vi "CreateImages.vi"(8 "error in (no error)":errorcluster) -> (0 "error out":errorcluster, 3 "Images":T1)   [LabVIEW 2015]
uses:
  controls/Images.ctl
  <vilib>/vision/Image Controls.llb/IMAQ Image.ctl
  <vilib>/vision/NI_Vision_Development_Module.lvlib
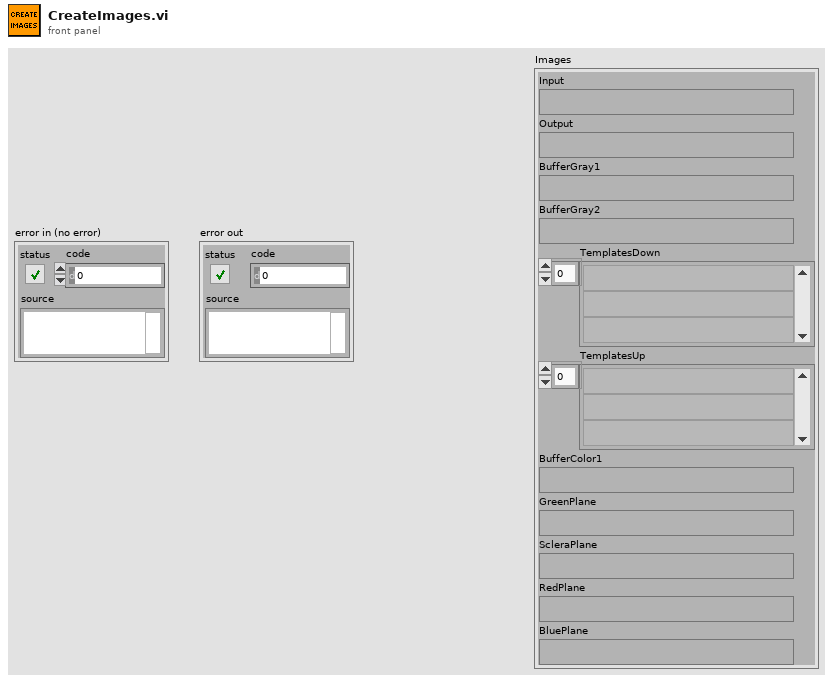
[diagram p1: front panel]
types:
  T1 = typedef "Images.ctl" = cluster{"Input":T2, "Output":T2, "BufferGray1":T2, "BufferGray2":T2, "TemplatesDown":T2[], "TemplatesUp":T2[], "BufferColor1":T2, "GreenPlane":T2, "ScleraPlane":T2, "RedPlane":T2, "BluePlane":T2}
  T2 = typedef "IMAQ Image.ctl" = refnum<image>
  T3 = typedef "Image Type" = u32
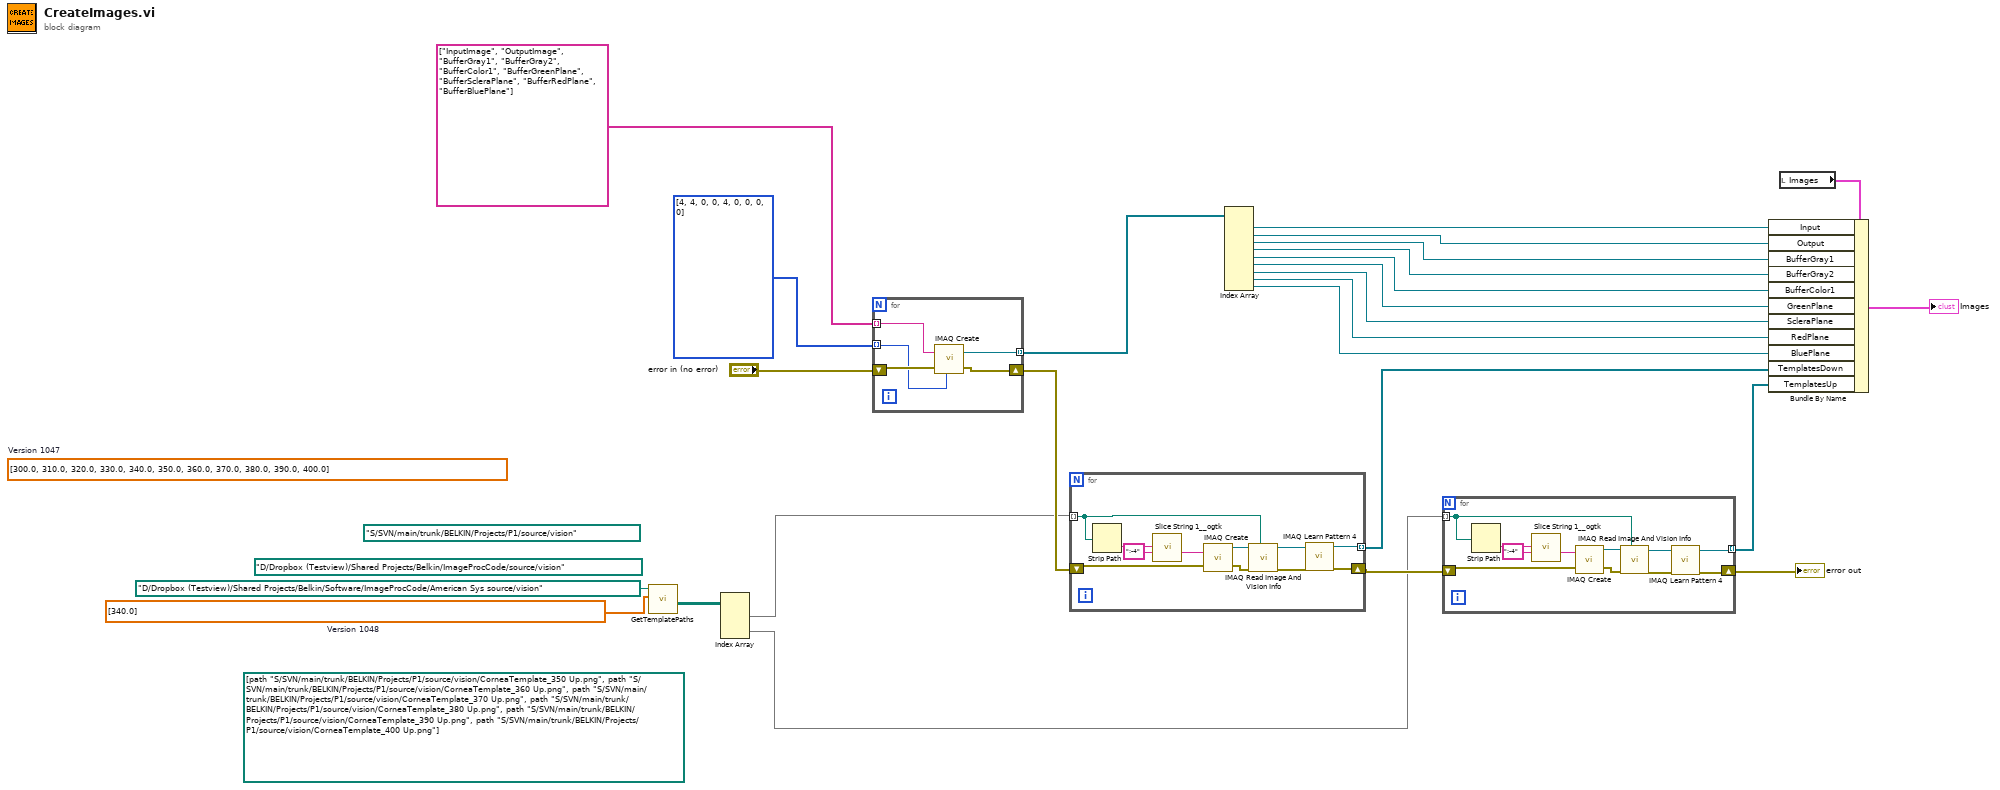
[diagram p0: block diagram]
diagram:
  (unwired) path "D:/Dropbox (Testview)/Shared Projects/Belkin/ImageProcCode/source/vision" ("Folder")
  (unwired) path "S:/SVN/main/trunk/BELKIN/Projects/P1/source/vision" ("Folder")
  (unwired) dbl[] [300.0, 310.0, 320.0, 330.0, 340.0, 350.0, 360.0, 370.0, 380.0, 390.0, 400.0]  # Version 1047
  w4 = dbl[] [340.0]  # Version 1048
  w17 = T3[] [4, 4, 0, 0, 4, 0, 0, 0, 0] items=["Grayscale (U8)", "Grayscale (I16)", "Grayscale (SGL)", "Complex (CSG)", "RGB (U32)", "HSL (U32)", "RGB (U64)", "Grayscale (U16)"]
  (unwired) path[] [path "S:/SVN/main/trunk/BELKIN/Projects/P1/source/vision/CorneaTemplate_350 Up.png", path "S:/SVN/main/trunk/BELKIN/Projects/P1/source/vision/CorneaTemplate_360 Up.png", path "S:/SVN/main/trunk/BELKIN/Projects/P1/source/vision/CorneaTemplate_370 Up.png", path "S:/SVN/main/trunk/BELKIN/Projects/P1/source/vision/CorneaTemplate_380 Up.png", path "S:/SVN/main/trunk/BELKIN/Projects/P1/source/vision/CorneaTemplate_390 Up.png", path "S:/SVN/main/trunk/BELKIN/Projects/P1/source/vision/CorneaTemplate_400 Up.png"]
  n1 = call "GetTemplatePaths.vi"("Diameters"=w4, "Folder"=path "D:/Dropbox (Testview)/Shared Projects/Belkin/Software/ImageProcCode/American Sys source/vision") -> ("Templates 2D"=w9:path[][])  [unwired: 6 in, 3 out]
  n2 = Index Array(array=w9) -> (element #1=w8:path[], element #2=w7:path[])  [unwired: 4 in]
  n3 = for {
    tunnel: string[] ["InputImage", "OutputImage", "BufferGray1", "BufferGray2", "BufferColor1", "BufferGreenPlane", "BufferScleraPlane", "BufferRedPlane", "BufferBluePlane"] -> [w29] mode=indexing
    shift-right: [w27] -> w10
    shift-left: "error in (no error)" -> [w30]
    tunnel: w17 -> [w28] mode=indexing
    tunnel: [w26] -> w16 mode=indexing
    n4 = call "IMAQ Create"("Image Name"=w29, "Image Type"=w28, "error in (no error)"=w30) -> ("New Image"=w26:T2, "error out"=w27:errorcluster)  [unwired: 1 in, 1 out]
  }
  n5 = for {
    tunnel: [w37] -> w23 mode=indexing
    tunnel: w8 -> [w34] mode=indexing
    shift-right: [w35] -> w22
    shift-left: w10 -> [w40]
    n6 = Strip Path(path=w34) -> (name=w32:string)  [unwired: 1 out]
    n7 = call <userlib>:"Slice String 1__ogtk.vi"("Subset (i:j)"=":-4", "String"=w32) -> ("Substring (String[i:j])"=w33:string)  [unwired: 7 in]
    n8 = call "IMAQ Create"("Image Name"=w33, "error in (no error)"=w40) -> ("New Image"=w41:T2, "error out"=w39:errorcluster)  [unwired: 2 in, 1 out]
    n9 = call "IMAQ Read Image And Vision Info"("File Path"=w34, "error in (no error)"=w39, "Image"=w41) -> ("error out"=w36:errorcluster, "Image Out"=w38:T2)  [unwired: 1 in, 6 out]
    n10 = call "IMAQ Learn Pattern 4"("error in (no error)"=w36, "Image"=w38) -> ("error out"=w35:errorcluster, "Template Image Out"=w37:T2)  [unwired: 7 in, 1 out]
  }
  n11 = Index Array(array=w16) -> (element #1=w15:T2, element #2=w14:T2, element #3=w13:T2, element #4=w12:T2, element #5=w11:T2, element #6=w5:T2, element #7=w3:T2, element #8=w2:T2, element #9=w1:T2)  [unwired: 9 in]
  n12 = for {
    tunnel: [w47] -> w20 mode=indexing
    tunnel: w7 -> [w42] mode=indexing
    shift-right: [w46] -> w21
    shift-left: w22 -> [w51]
    n13 = Strip Path(path=w42) -> (name=w44:string)  [unwired: 1 out]
    n14 = call <userlib>:"Slice String 1__ogtk.vi"("Subset (i:j)"=":-4", "String"=w44) -> ("Substring (String[i:j])"=w43:string)  [unwired: 7 in]
    n15 = call "IMAQ Create"("Image Name"=w43, "error in (no error)"=w51) -> ("New Image"=w52:T2, "error out"=w50:errorcluster)  [unwired: 2 in, 1 out]
    n16 = call "IMAQ Read Image And Vision Info"("File Path"=w42, "error in (no error)"=w50, "Image"=w52) -> ("error out"=w48:errorcluster, "Image Out"=w49:T2)  [unwired: 1 in, 6 out]
    n17 = call "IMAQ Learn Pattern 4"("error in (no error)"=w48, "Image"=w49) -> ("error out"=w46:errorcluster, "Template Image Out"=w47:T2)  [unwired: 7 in, 1 out]
  }
  "error out" <- w21
  n18 = local read "Images"() -> (w24:T1)
  n19 = Bundle By Name(cluster=w24, "Input"=w15, "Output"=w14, "BufferGray1"=w13, "BufferGray2"=w12, "BufferColor1"=w11, "GreenPlane"=w5, "ScleraPlane"=w3, "RedPlane"=w2, "BluePlane"=w1, "TemplatesDown"=w23, "TemplatesUp"=w20) -> (→"Images":T1)
